vi "Linearly Resample Time Series Data.vi"(10 "Duration (s)":i32, 11 "Irregular Data":dbl[][](array[numeric])) -> (3 "Regular Data":dbl[][](array[numeric]))   [LabVIEW 2013, in "Data Log Fetcher.lvlib"]
uses:
  Data Log Fetcher.lvlib
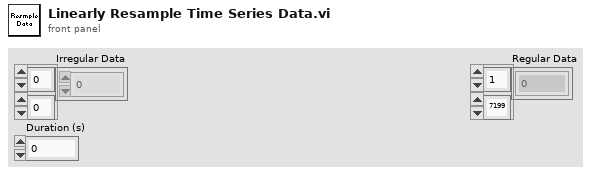
[diagram p1: front panel]
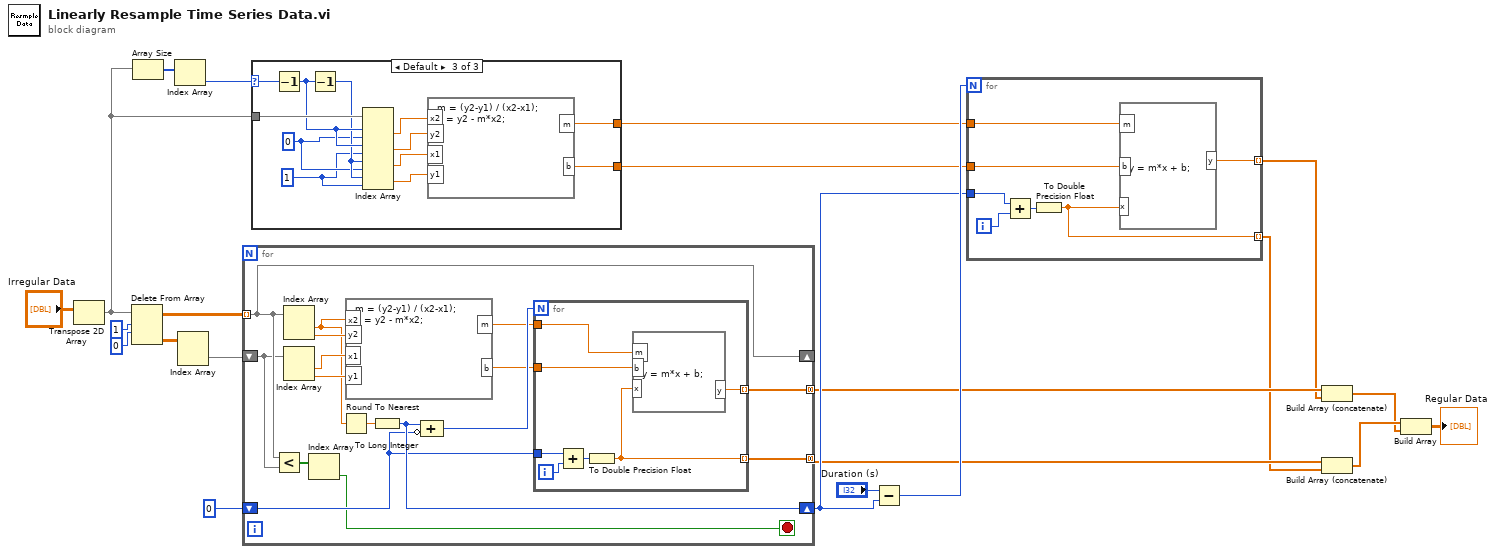
[diagram p0: block diagram]
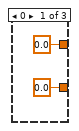
[diagram p2: hidden frame]
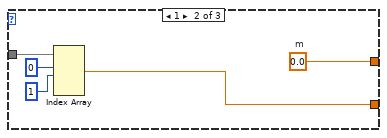
[diagram p3: hidden frame]
diagram:
  n1 = Transpose 2D Array(2D array="Irregular Data") -> (transposed array=w11:dbl[][])
  n2 = Delete From Array(array=w11, length=1, index (row)=0 ("disabled index (col)")) -> (deleted portion=w17:dbl[][], array with subset deleted=w18:dbl[][])  [unwired: 1 in]
  n3 = Array Size(array=w11) -> (size(s)=w14:i32[])
  n4 = Index Array(array=w14) -> (element=w13:i32)  [unwired: 1 in]
  n5 = Index Array(array=w17) -> (element=w16:dbl[])  [unwired: 2 in]
  n6 = for {
    tunnel: w18 -> [w25] mode=indexing
    shift-right: [w25] -> _
    shift-left: w16 -> [w24]
    shift-right: [w33] -> w9
    shift-left: 0 ("dimension size") -> [w31]
    tunnel: [w28] -> w6 mode=concatenating
    tunnel: [w27] -> w5 mode=concatenating
    stop <- w23 stop-if-true
    n7 = Less?(x=w25, y=w24) -> (x < y?=w26:bool[])
    n8 = Index Array(array=w25) -> (element #1=w35:dbl, element #2=w38:dbl)  [unwired: 2 in]
    n9 = Index Array(array=w24) -> (element #1=w37:dbl, element #2=w36:dbl)  [unwired: 2 in]
    n10 = Index Array(array=w26) -> (element=w23:bool)  [unwired: 1 in]
    n11 = Round To Nearest(number=w35) -> (nearest integer value=w34:dbl)
    n12 = formula code="m = (y2-y1) / (x2-x1);\nb = y2 - m*x2;"("x1"=w37, "y1"=w36, "x2"=w35, "y2"=w38) -> ("m"=w30:dbl, "b"=w29:dbl)
    n13 = To Long Integer(number=w34) -> (32bit integer=w33:i32)
    n14 = Compound Arithmetic op=ADD(w33, invert w31) -> (w32:i32)
    n15 = for {
      N: w32 -> [_]
      tunnel: w31 -> [w45]
      tunnel: w30 -> [w43]
      tunnel: w29 -> [w42]
      tunnel: [w40] -> w28 mode=indexing
      tunnel: [w39] -> w27 mode=indexing
      i -> [w44]
      n16 = Add(x=w45, y=w44) -> (x+y=w41:i32)
      n17 = To Double Precision Float(number=w41) -> (double precision float=w39:dbl)
      n18 = formula code="y = m*x + b;"("x"=w39, "m"=w43, "b"=w42) -> ("y"=w40:dbl)
    }
  }
  n19 = case shown="Default" w13 {
    selector: w13 -> [_ _ w64]
    tunnel: w11 -> [_ w52 w63]
    tunnel: [0.0 ("m") w50 w54] -> w8
    tunnel: [0.0 ("b") w48 w53] -> w7
    frame 0 {
    }
    frame 1 {
      w50 = 0.0  # m
      n20 = Index Array(array=w52, index (row) #1=0 ("index (row)"), index (col) #1=1 ("disabled index (col)")) -> (element #1=w48:dbl)  [unwired: 2 in, 1 out]
    }
    frame Default {
      w60 = 0 ("disabled index (col)")
      w59 = 1 ("disabled index (col)")
      n21 = Decrement(x=w64) -> (x-1=w62:i32)
      n22 = Decrement(x=w62) -> (x-1=w61:i32)
      n23 = Index Array(array=w63, index (row) #1=w62, index (col) #1=w60, index (row) #2=w62, index (col) #2=w59, index (row) #3=w61, index (col) #3=w60, index (row) #4=w61, index (col) #4=w59) -> (element #1=w58:dbl, element #2=w57:dbl, element #3=w56:dbl, element #4=w55:dbl)
      n24 = formula code="m = (y2-y1) / (x2-x1);\nb = y2 - m*x2;"("x1"=w56, "y1"=w55, "x2"=w58, "y2"=w57) -> ("m"=w54:dbl, "b"=w53:dbl)
    }
  }
  n25 = Subtract(x="Duration (s)", y=w9) -> (x-y=w10:i32)
  n26 = for {
    N: w10 -> [_]
    tunnel: w9 -> [w70]
    tunnel: w8 -> [w68]
    tunnel: w7 -> [w67]
    tunnel: [w66] -> w3 mode=indexing
    tunnel: [w65] -> w4 mode=indexing
    i -> [w71]
    n27 = Add(x=w70, y=w71) -> (x+y=w69:i32)
    n28 = To Double Precision Float(number=w69) -> (double precision float=w66:dbl)
    n29 = formula code="y = m*x + b;"("x"=w66, "m"=w68, "b"=w67) -> ("y"=w65:dbl)
  }
  n30 = Build Array (concatenate)(w6, w4) -> (w1:dbl[])
  n31 = Build Array (concatenate)(w5, w3) -> (w2:dbl[])
  n32 = Build Array(w2, w1) -> (→"Regular Data":dbl[][])
